vi "Arm_Controller.vi"(8 "error in (no error)":errorcluster) -> (0 "error out":errorcluster, 3 "Arm Counter":dbl, 4 "Arm Controller":bool)   [LabVIEW 2014]
uses:
  Start.vi
  <userlib>/UCSD Robotics Lab/Robotics-Cape/LV/libroboticscape.lvlib
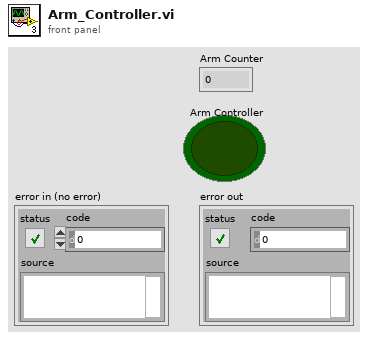
[diagram p1: front panel]
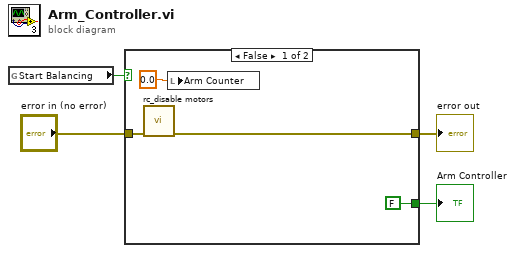
[diagram p0: block diagram]
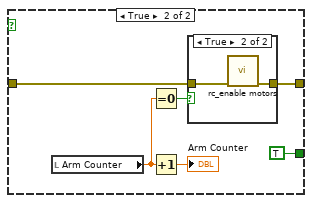
[diagram p2: hidden frame]
diagram:
  n1 = global read "Start.vi" "Start Balancing"() -> (w1:bool)
  n2 = case shown="False" w1 {
    tunnel: "error in (no error)" -> [w8 w14]
    tunnel: [w7 w13] -> w4
    tunnel: [FALSE ("Arm Controller") TRUE ("Arm Controller")] -> w2
    frame False {
      n3 = call <userlib>:"rc_disable motors.vi"("error in (no error)"=w8) -> ("error out"=w7:errorcluster)  [unwired: 9 in, 1 out]
      n4 = local write "Arm Counter"(0.0 ("Arm Counter")) -> ()
    }
    frame True {
      n5 = local read "Arm Counter"() -> (w9:dbl)
      n6 = Equal To 0?(x=w9) -> (x = 0?=w11:bool)
      n7 = Increment(x=w9) -> (x+1=→"Arm Counter":dbl)
      n8 = case shown="True" w11 {
        tunnel: w14 -> [w15 w17]
        tunnel: [w15 w16] -> w13
        frame False {
        }
        frame True {
          n9 = call <userlib>:"rc_enable motors.vi"("error in (no error)"=w17) -> ("error out"=w16:errorcluster)  [unwired: 9 in, 1 out]
        }
      }
    }
  }
  "error out" <- w4
  "Arm Controller" <- w2
